vi "Log Test Results.vi"(8 "error in":errorcluster, 11 "TDMS in":refnum<class "TDMS.lvclass">) -> (0 "error out":errorcluster, 3 "TDMS out":refnum<class "TDMS.lvclass">)   [LabVIEW 2019, in "TDMS.lvlib" / "TDMS.lvclass"]
uses:
  TDMS.lvclass
  TDMS.lvclass/TDMS.ctl
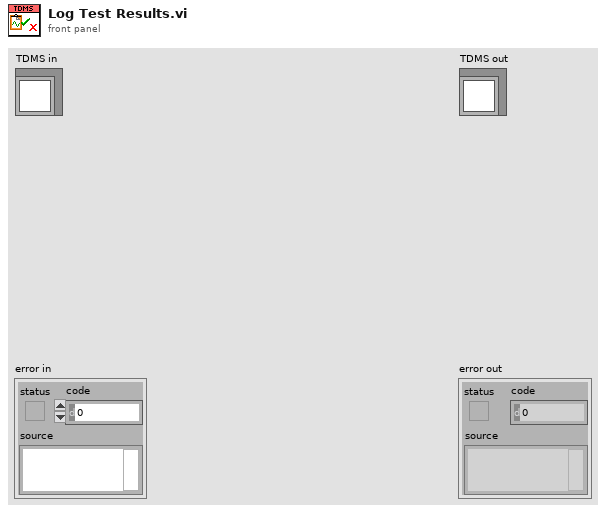
[diagram p1: front panel]
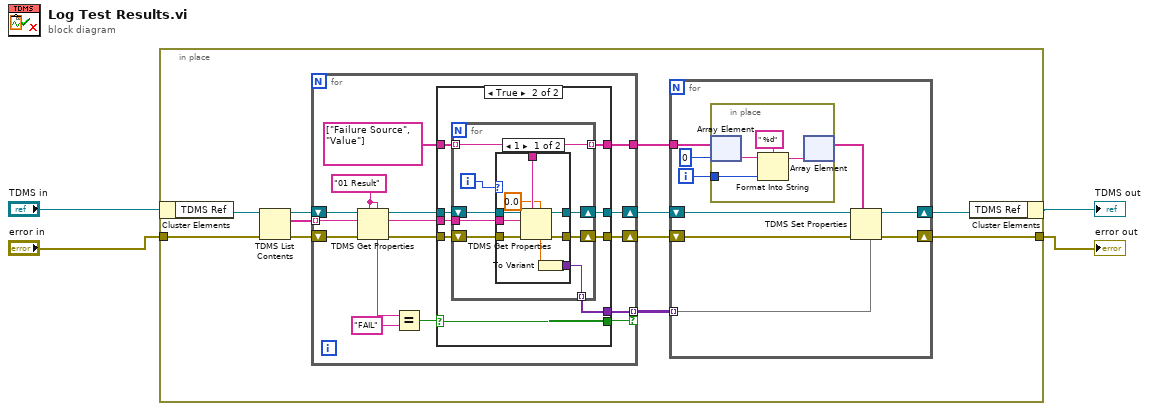
[diagram p0: block diagram]
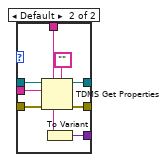
[diagram p3: hidden frame]
diagram:
  n1 = in-place {
    in-place-border: "error in" -> [w6]
    in-place-border: [w5] -> w1
    n2 = in-place-cluster #1("TDMS in") -> ("TDMS Ref"=w15:refnum<k34>)
    n3 = TDMS List Contents(4:w6, 7:w15) -> (0:w12:errorcluster, 2:w14:string[], 3:w13:refnum<k34>)  [unwired: 1 in, 1 out]
    n4 = for {
      tunnel: w14 -> [w42] mode=indexing
      shift-right: [w35] -> w10
      shift-left: w13 -> [w44]
      shift-right: [w34] -> w9
      shift-left: w12 -> [w41]
      tunnel: [w33] -> w8 mode=indexing if=w32
      tunnel: [w29] -> w11
      w43 = "01 Result" ("property name")
      n5 = TDMS Get Properties(5:w43, 7:w43, 8:w41, 10:w42, 11:w44) -> (0:w36:errorcluster, 2:w30:string, 3:w37:refnum<k34>, 4:w40:string)  [unwired: 1 in, 2 out]
      n6 = Equal?(x=w40, y="FAIL") -> (x = y?=w38:bool)
      n7 = case shown="True" w38 {
        selector: w38 -> [_ w51]
        tunnel: w37 -> [w47 w55]
        tunnel: w36 -> [w46 w56]
        tunnel: [w47 w54] -> w35
        tunnel: [w46 w53] -> w34
        tunnel: [_ w52] -> w33
        tunnel: [_ w51] -> w32
        tunnel: string[] ["Failure Source", "Value"] -> [w45 w49]
        tunnel: w30 -> [_ w50]
        tunnel: [w45 w48] -> w29
        frame False {
        }
        frame True {
          n8 = for {
            tunnel: [w60] -> w52 mode=indexing
            tunnel: w50 -> [w59]
            shift-right: [w61] -> w53
            shift-left: w56 -> [w64]
            shift-right: [w62] -> w54
            shift-left: w55 -> [w63]
            tunnel: w49 -> [w58] mode=indexing
            tunnel: [w58] -> w48 mode=indexing
            i -> [w57]
            n9 = case shown="1" w57 {
              tunnel: w64 -> [w73 w82]
              tunnel: w63 -> [w72 w81]
              tunnel: [w71 w80] -> w62
              tunnel: [w70 w79] -> w61
              tunnel: [w65 w74] -> w60
              tunnel: w59 -> [w68 w77]
              tunnel: w58 -> [w67 w76]
              frame 1 {
                n10 = TDMS Get Properties(5:0.0, 7:w67, 8:w73, 10:w68, 11:w72) -> (0:w70:errorcluster, 3:w71:refnum<k34>, 4:w69:dbl)  [unwired: 1 in, 3 out]
                n11 = To Variant(anything=w69) -> (Variant=w65:variant)
              }
              frame Default {
                n12 = TDMS Get Properties(5:"", 7:w76, 8:w82, 10:w77, 11:w81) -> (0:w79:errorcluster, 3:w80:refnum<k34>, 4:w78:string)  [unwired: 1 in, 3 out]
                n13 = To Variant(anything=w78) -> (Variant=w74:variant)
              }
            }
          }
        }
      }
    }
    n14 = for {
      tunnel: w11 -> [w19]
      shift-right: [w21] -> w7
      shift-left: w10 -> [w22]
      shift-right: [w24] -> w5
      shift-left: w9 -> [w23]
      tunnel: w8 -> [w20] mode=indexing
      i -> [w16]
      n15 = in-place {
        in-place-border: w16 -> [w27]
        n16 = in-place-array #2(w19, 0) -> (w28:string)
        n17 = Format Into String(format string=" %d", initial string=w28, w27) -> (resulting string=w25:string)  [unwired: 1 in, 1 out]
        n18 = in-place-array #2(w25) -> (w17:string[])  [unwired: 1 out]
      }
      n19 = TDMS Set Properties(5:w20, 7:w17, 8:w23, 11:w22) -> (0:w24:errorcluster, 3:w21:refnum<k34>)  [unwired: 2 in, 2 out]
    }
    n20 = in-place-cluster #1("TDMS Ref"=w7) -> (→"TDMS out":refnum<class "TDMS.lvclass">)
  }
  "error out" <- w1
